vi "Moving Motor.vi"() -> ()   [LabVIEW 2016]
uses:
  <vilib>/NXT/Block Support/NXT_InputPort.ctl
  <vilib>/NXT/Block Support/NXT_OutputPort.ctl
  <vilib>/NXT/Dual Mode Library/Sensors/Touch_Pressed.vi
  <vilib>/NXT/NXTIO Xnodes/NXTIONodeSubVIs/LEGOStopAllMotors.vi
  <vilib>/NXT/NXTIO Xnodes/NXTIONodeSubVIs/NXTMoveMotors.vi
  <vilib>/NXT/NXTIO Xnodes/NXTIOXNode/NXTIO.xnode
  <vilib>/NXT/Subs/LVHSConnector.ctl
  <vilib>/NXT/NXTIO Xnodes/AddressXNode/NXTIOAddress.xnode
  <vilib>/NXT/LegoClasses/BrickReference/BrickReference.lvclass
panel:
  in  "stop":bool
  out "Press":bool
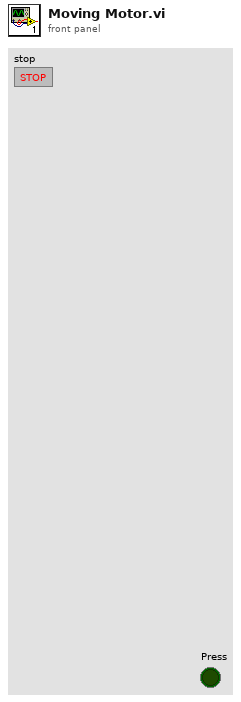
[diagram p1: front panel]
types:
  T1 = typedef "NXT_InputPort.ctl" = u32
  T2 = typedef "LVHSConnector.ctl" = refnum<class "BrickReference.lvclass">
  T3 = typedef "NXT_OutputPort.ctl" = u8
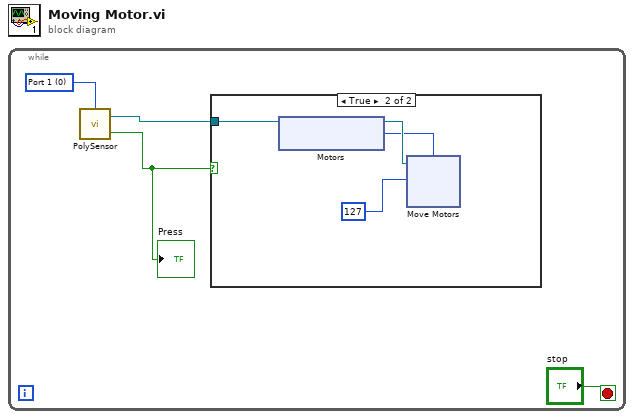
[diagram p0: block diagram]
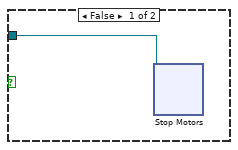
[diagram p2: hidden frame]
diagram:
  n1 = while {
    stop <- "stop" stop-if-true
    w4 = T1 0 items=["Port 1", "Port 2", "Port 3", "Port 4"] ("Port (Port 1)")
    n2 = call-poly <vilib>:"PolySensor.vi"("Port (Port 1)"=w4) -> ("Yes / No"=w3:bool, "NXT/EV3"=w2:T2)  [unwired: 2 in]
    "Press" <- w3
    n3 = case shown="True" w3 {
      tunnel: w2 -> [w5 w11]
      frame False {
        n4 = xnode "Stop Motors"("NXT/EV3"=w5) -> ()  [unwired: 1 in, 1 out]
      }
      frame True {
        n5 = xnode "Motors"() -> ("Motor"=w9:T3)
        n6 = xnode "Move Motors"("Power/Speed 1"=i8 127, "Motors"=w9, "NXT/EV3"=w11) -> ()  [unwired: 1 out]
      }
    }
  }
